vi "EventDrivenQSM-Enum.vi"() -> ()   [LabVIEW 2020]
uses:
  EventDrivenQSM-State.ctl
panel:
  in  "Cmd":bool
  in  "Exit":bool
  out "error out":errorcluster
  in  "error in":errorcluster
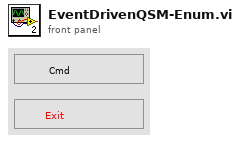
[diagram p1: front panel]
types:
  T1 = typedef "EventDrivenQSM-State.ctl" = enum16{"IDLE", "----------- CMD -----------", "CMD:Init", "CMD:Exit", "----------- CORE -----------", "CORE:Error", "CORE:Exit", "----------- DATA -----------", "DATA:Init", "DATA:Cleanup", "----------- GUI -----------", "GUI:Init", "GUI:SetMenu", "GUI:SetCusor", "GUI:FP", "----------- RESERVED -----------"}
  T2 = cluster{"Current VI Reference":refnum<vi>, "Close Panel on Exit?":bool}
  T3 = cluster{"Core":cluster{"Current VI Reference":refnum<vi>, "Close Panel on Exit?":bool}, "Your Boolean data":bool, "Your string data":string}
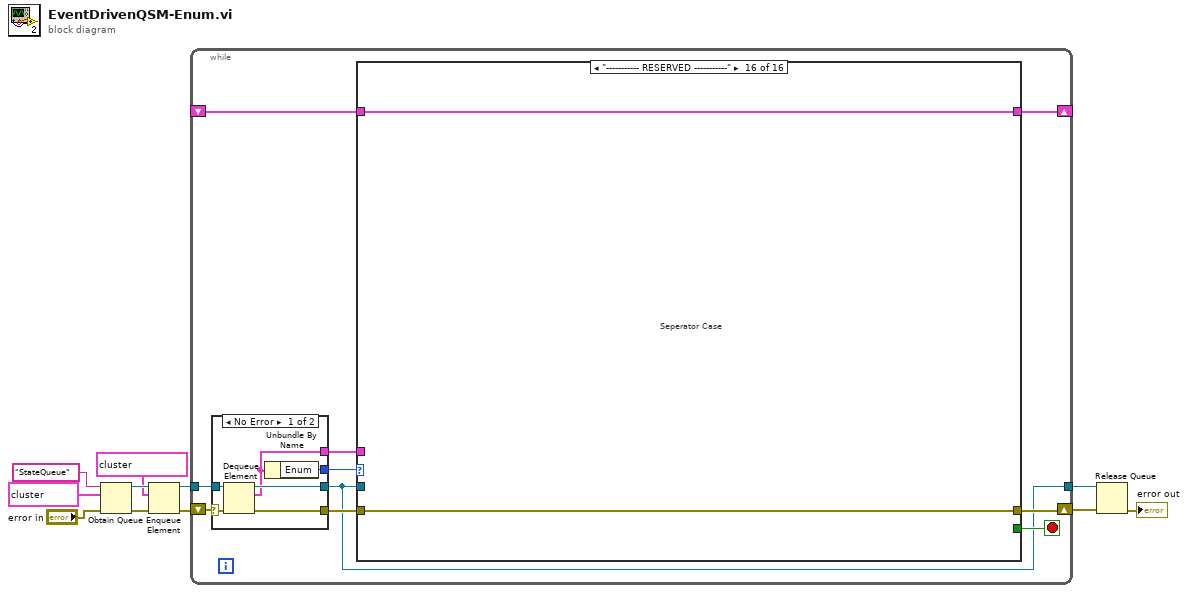
[diagram p0: block diagram]
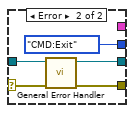
[diagram p2: hidden frame]
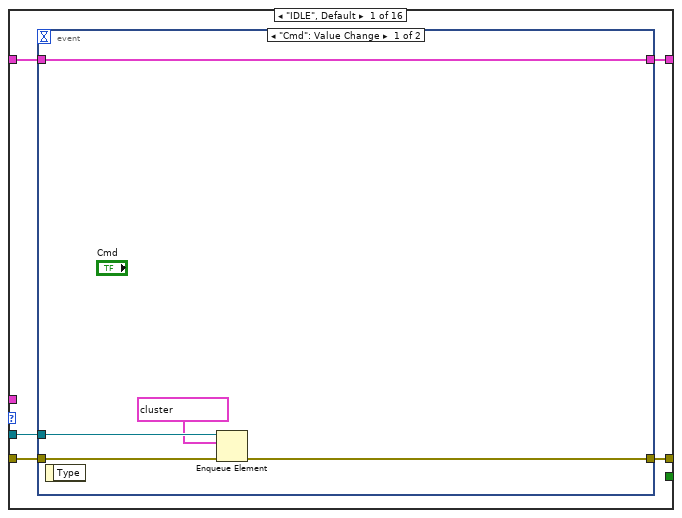
[diagram p3: hidden frame]
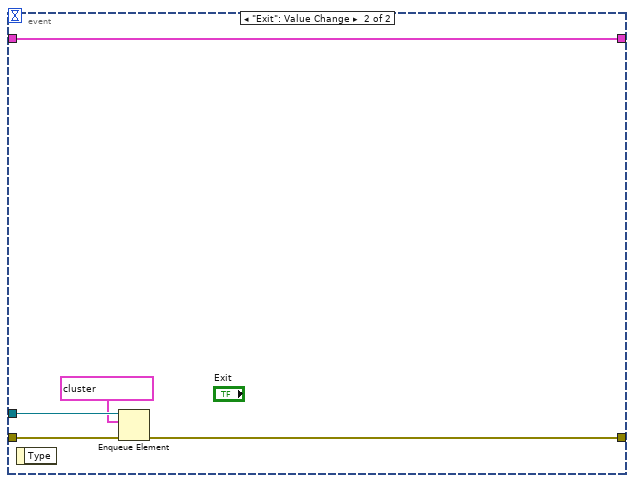
[diagram p4: hidden frame]
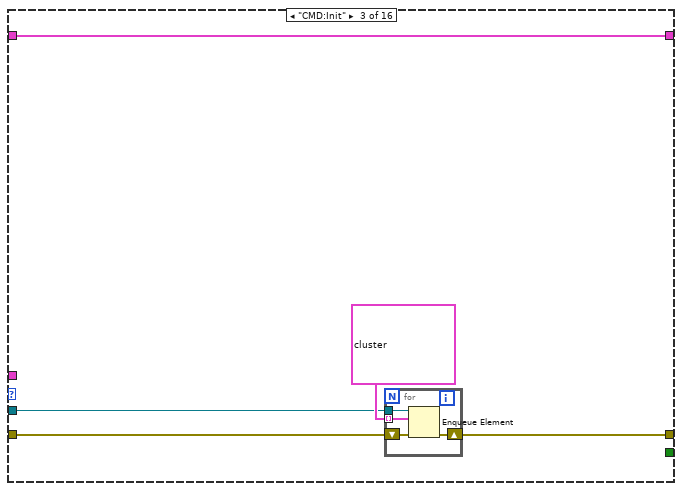
[diagram p6: hidden frame]
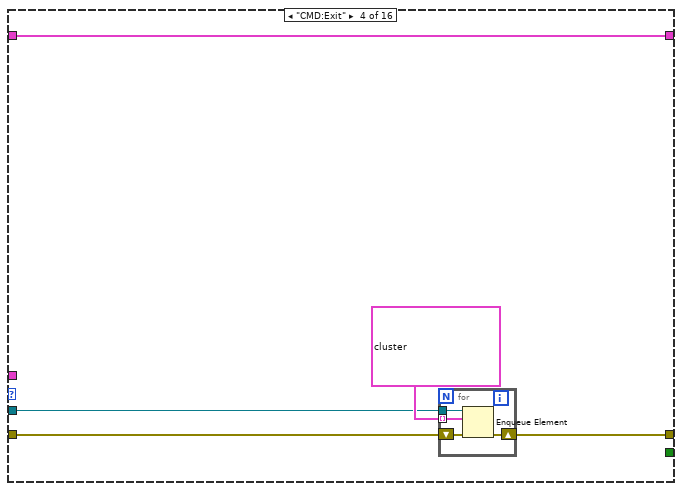
[diagram p7: hidden frame]
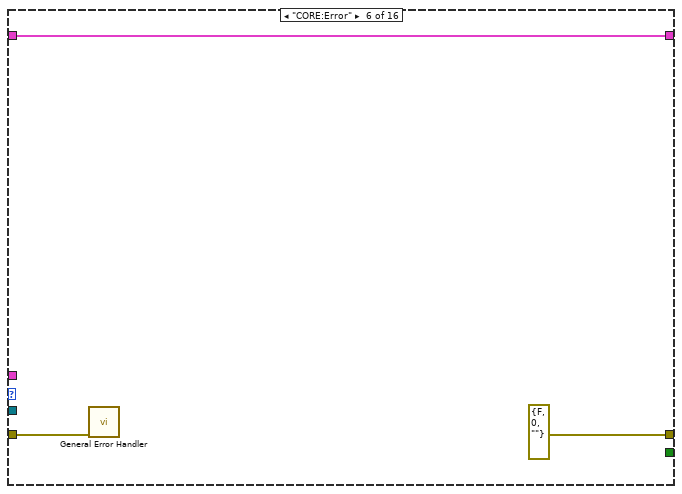
[diagram p9: hidden frame]
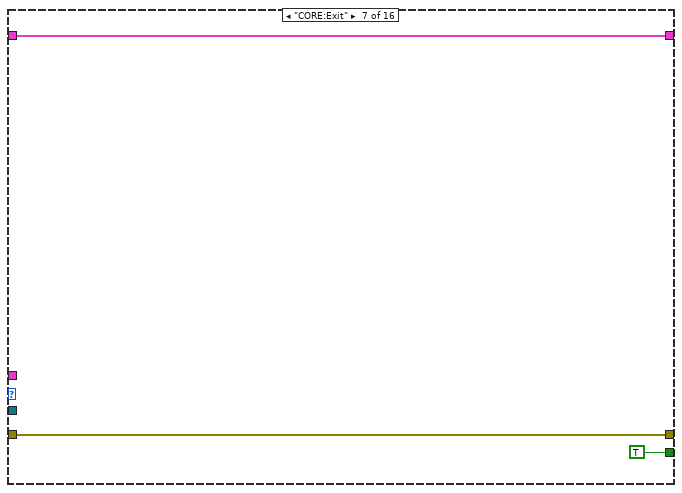
[diagram p10: hidden frame]
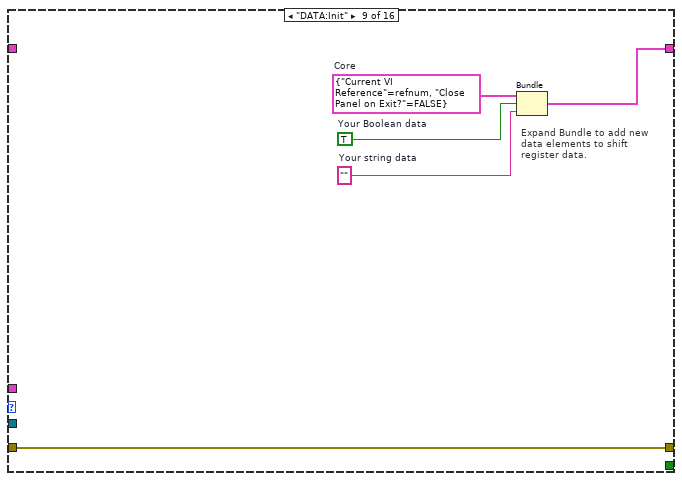
[diagram p12: hidden frame]
diagram:
  n1 = Obtain Queue(name (unnamed)="StateQueue", element data type=cluster{"Data":variant, "Enum":T1} {"Data"=variant, "Enum"=enum."IDLE"} ("Queue Data"), error in (no error)="error in") -> (queue out=w10:refnum<queue>, error out=w9:errorcluster)  [unwired: 2 in, 1 out]
  n2 = Enqueue Element(queue=w10, element=cluster{"Data":variant, "Enum":T1} {"Data"=variant, "Enum"=enum."CMD:Init"} ("Queue Data"), error in (no error)=w9) -> (queue out=w4:refnum<queue>, error out=w3:errorcluster)  [unwired: 1 in, 1 out]
  n3 = while {
    shift-right: [w20] -> w8
    shift-left: w3 -> [w18]
    tunnel: w4 -> [w19]
    tunnel: [w16] -> w7
    shift-right: [w15] -> _
    shift-left: _ -> [w12]
    stop <- w21 stop-if-true
    n4 = case shown="No Error" w18 {
      selector: w18 -> [w26 w31]
      tunnel: w19 -> [w27 w30]
      tunnel: [w25 w30] -> w16
      tunnel: [w24 w29] -> w17
      tunnel: [w23 EventDrivenQSM-State."CMD:Exit" ("Enum")] -> w14
      tunnel: [w22 _] -> w13
      frame No Error {
        n5 = Dequeue Element(queue=w27, error in (no error)=w26) -> (queue out=w25:refnum<queue>, element=w22:cluster{"Data":variant, "Enum":T1}, error out=w24:errorcluster)  [unwired: 1 in, 1 out]
        n6 = Unbundle By Name(w22) -> ("Enum"=w23:T1)
      }
      frame Error {
        n7 = call <vilib>:"General Error Handler.vi"("error in (no error)"=w31) -> ("error out"=w29:errorcluster)  [unwired: 10 in, 4 out]
      }
    }
    n8 = case shown="\"----------- RESERVED -----------\"" w14 {
      tunnel: [_ _ _ _ _ _ TRUE _ _ _ _ _ _ _ _ _] -> w21
      tunnel: w17 -> [w36 w48 w53 w61 w68 w71 w73 w76 w77 w83 w85 w87 w89 w91 w93 w95]
      tunnel: [w34 w48 w52 w60 w68 errorcluster {"status"=FALSE, "code"=0, "source"=""} ("error out") w73 w76 w77 w83 w85 w87 w89 w91 w93 w95] -> w20
      tunnel: w16 -> [w35 _ w50 w59 _ _ _ _ _ _ _ _ _ _ _ _]
      tunnel: [w32 w47 w49 w58 w67 w69 w72 w75 w79 w82 w84 w86 w88 w90 w92 w94] -> w15
      tunnel: w13 -> [_ _ _ _ _ _ _ _ _ _ _ _ _ _ _ _]
      tunnel: w12 -> [w33 w47 w49 w58 w67 w69 w72 w75 _ w82 w84 w86 w88 w90 w92 w94]
      frame "IDLE", Default {
        n9 = event shown="[0] \"Cmd\": Value Change" {
          selector: _ -> [_ _]
          dyn-events: _ -> [_ _]
          timeout: _ -> [_ _]
          tunnel: w36 -> [w41 w45]
          tunnel: w35 -> [w40 w46]
          tunnel: [w39 w44] -> w34
          tunnel: [w38 w42] -> w32
          tunnel: w33 -> [w38 w42]
          event "Cmd": Value Change {
            n10 = event-data() -> ()  [unwired: 1 in, 1 out]
            n11 = Enqueue Element(queue=w40, element=cluster{"Data":variant, "Enum":T1} {"Data"=variant, "Enum"=enum."CMD:Init"} ("Queue Data"), error in (no error)=w41) -> (error out=w39:errorcluster)  [unwired: 1 in, 2 out]
          }
          event "Exit": Value Change {
            n12 = event-data() -> ()  [unwired: 1 in, 1 out]
            n13 = Enqueue Element(queue=w46, element=cluster{"Data":variant, "Enum":T1} {"Data"=variant, "Enum"=enum."CMD:Exit"} ("Queue Data"), error in (no error)=w45) -> (error out=w44:errorcluster)  [unwired: 1 in, 2 out]
          }
        }
      }
      frame "----------- CMD -----------" {
        # "Seperator Case"
      }
      frame "CMD:Init" {
        n14 = for {
          tunnel: w50 -> [w55]
          shift-right: [w56] -> w52
          shift-left: w53 -> [w57]
          tunnel: cluster{"Data":variant, "Enum":T1}[] [{"Data"=variant, "Enum"=enum."DATA:Init"}, {"Data"=variant, "Enum"=enum."GUI:Init"}, {"Data"=variant, "Enum"=enum."IDLE"}] -> [w54] mode=indexing
          n15 = Enqueue Element(queue=w55, element=w54, error in (no error)=w57) -> (error out=w56:errorcluster)  [unwired: 1 in, 2 out]
        }
      }
      frame "CMD:Exit" {
        n16 = for {
          tunnel: w59 -> [w64]
          shift-right: [w65] -> w60
          shift-left: w61 -> [w66]
          tunnel: cluster{"Data":variant, "Enum":T1}[] [{"Data"=variant, "Enum"=enum."GUI:FP"}, {"Data"=variant, "Enum"=enum."DATA:Cleanup"}, {"Data"=variant, "Enum"=enum."CORE:Exit"}, {"Data"=variant, "Enum"=enum."IDLE"}] -> [w63] mode=indexing
          n17 = Enqueue Element(queue=w64, element=w63, error in (no error)=w66) -> (error out=w65:errorcluster)  [unwired: 1 in, 2 out]
        }
      }
      frame "----------- CORE -----------" {
        # "Seperator Case"
      }
      frame "CORE:Error" {
        n18 = call <vilib>:"General Error Handler.vi"("error in (no error)"=w71) -> ()  [unwired: 10 in, 5 out]
      }
      frame "CORE:Exit" {
      }
      frame "----------- DATA -----------" {
        # "Seperator Case"
      }
      frame "DATA:Init" {
        w81 = T2 {"Current VI Reference"=refnum, "Close Panel on Exit?"=FALSE}  # Core
        w78 = ""  # Your string data
        w80 = TRUE  # Your Boolean data
        # "Expand Bundle to add new data elements to shift register data."
        n19 = Bundle("Core"=w81, "Your Boolean data"=w80, "Your string data"=w78) -> (w79:T3)  [unwired: 1 in]
      }
      frame "DATA:Cleanup" {
      }
      frame "----------- GUI -----------" {
        # "Seperator Case"
      }
      frame "GUI:Init" {
      }
      frame "GUI:SetMenu" {
      }
      frame "GUI:SetCusor" {
      }
      frame "GUI:FP" {
      }
      frame "----------- RESERVED -----------" {
        # "Seperator Case"
      }
    }
  }
  n20 = Release Queue(queue=w7, error in (no error)=w8) -> (error out=→"error out":errorcluster)  [unwired: 1 in, 2 out]
